vi "Device-Tester.vi"() -> ()   [LabVIEW 2011]
uses:
  <vilib>/Instr/_visa.llb/VISA Configure Serial Port (Instr).vi
panel:
  out "Bytes at Port":u32
  out "String Received":string
  in  "String to Send":string
  out "ExecTime":u32
  in  "BaudRate":u32(ring) items=["9600"=9600, "115200"=65535]
  in  "VISA resource name":refnum<visa-resource-name>
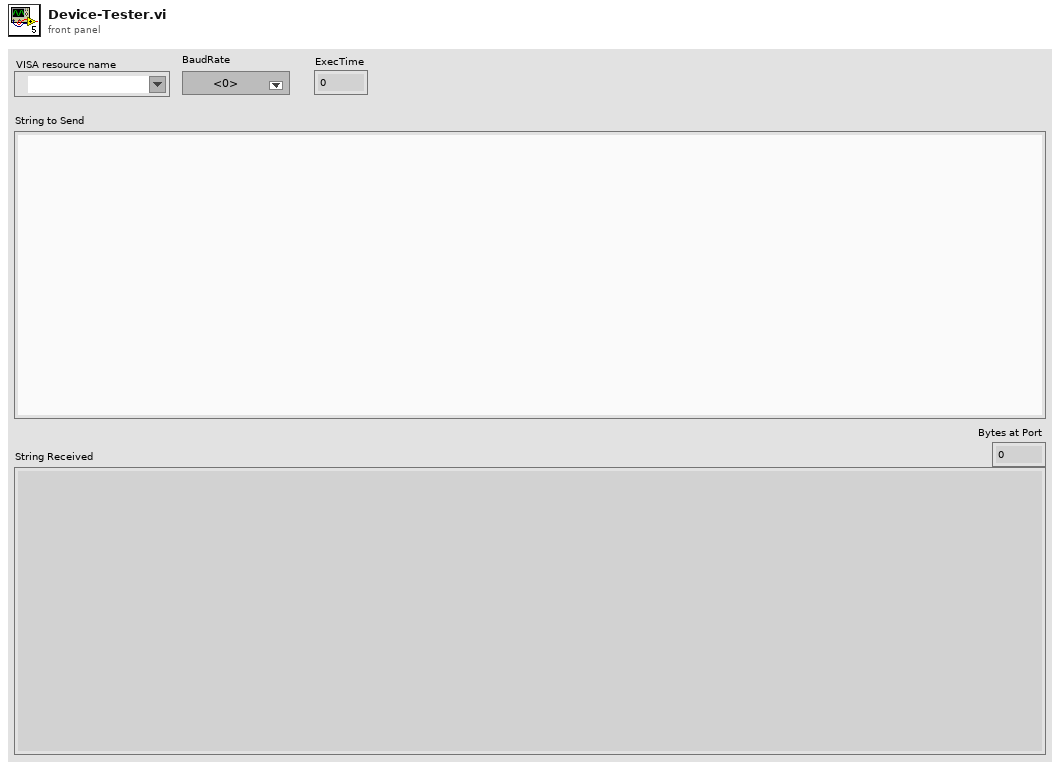
[diagram p1: front panel]
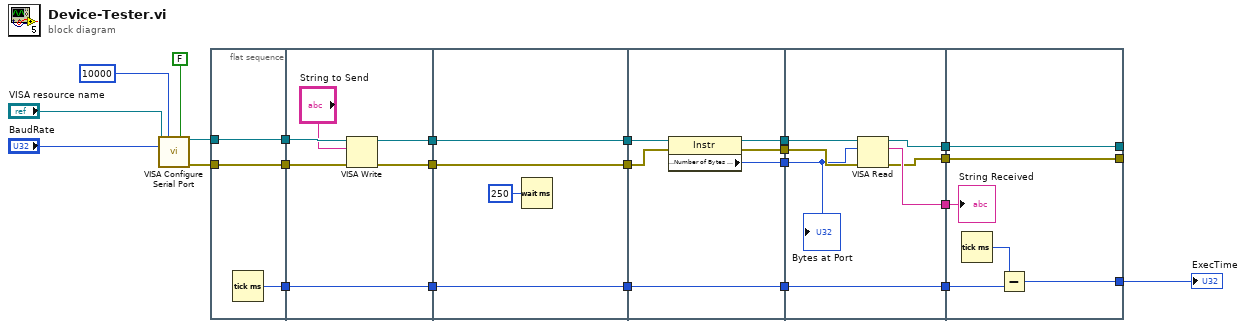
[diagram p0: block diagram]
diagram:
  n1 = call-poly "VISA Configure Serial Port"("VISA resource name"="VISA resource name", "timeout (10sec)"=u32 10000, "Enable Termination\nChar (T)"=FALSE ("Enable Termination\nChar (T)"), "baud rate (9600)"="BaudRate") -> ("VISA resource name out"=w20:refnum<visa-resource-name>, "error out"=w19:errorcluster)  [unwired: 10 in]
  n2 = flat-sequence {
    tunnel: w19 -> [w25]
    tunnel: w20 -> [w26]
    tunnel: [w26] -> w18
    tunnel: [w27] -> w17
    tunnel: [w25] -> w2
    tunnel: w18 -> [w32]
    tunnel: [w33] -> w9
    tunnel: w17 -> [w33]
    tunnel: [w30] -> w7
    tunnel: [w29] -> w5
    tunnel: w2 -> [w28]
    tunnel: w9 -> [w37]
    tunnel: [w37] -> w8
    tunnel: w7 -> [w36]
    tunnel: [w36] -> w6
    tunnel: w5 -> [w35]
    tunnel: [w35] -> w4
    tunnel: w8 -> [w43]
    tunnel: [w43] -> w12
    tunnel: w6 -> [w42]
    tunnel: w4 -> [w41]
    tunnel: [w40] -> w11
    tunnel: [w39] -> w10
    tunnel: [w38] -> w3
    tunnel: [w49] -> w16
    tunnel: [w44] -> w15
    tunnel: w12 -> [w50]
    tunnel: [w50] -> w14
    tunnel: [w45] -> w13
    tunnel: w11 -> [w48]
    tunnel: w10 -> [w47]
    tunnel: w3 -> [w46]
    tunnel: [w55] -> _
    tunnel: [w56] -> _
    tunnel: w16 -> [w56]
    tunnel: w15 -> [w55]
    tunnel: w14 -> [w53]
    tunnel: [w52] -> w1
    tunnel: w13 -> [w51]
    frame #0 {
      n3 = Tick Count (ms)() -> (millisecond timer value=w27:u32)
    }
    frame #1 {
      n4 = VISA Write(VISA resource name=w32, write buffer="String to Send", error in (no error)=w28) -> (VISA resource name out=w30:refnum<visa-resource-name>, error out=w29:errorcluster)  [unwired: 1 out]
    }
    frame #2 {
      n5 = Wait (ms)(milliseconds to wait=u32 250) -> ()  [unwired: 1 out]
    }
    frame #3 {
      n6 = property class="Instr"(reference=w42, error in=w41) -> (reference out=w40:refnum<visa-resource-name>, error out=w39:errorcluster, "Serial Settings:Number of Bytes at Serial Port"=w38:u32)
    }
    frame #4 {
      n7 = VISA Read(VISA resource name=w48, byte count=w46, error in (no error)=w47) -> (VISA resource name out=w49:refnum<visa-resource-name>, read buffer=w45:string, error out=w44:errorcluster)  [unwired: 1 out]
      "Bytes at Port" <- w46
    }
    frame #5 {
      n8 = Tick Count (ms)() -> (millisecond timer value=w54:u32)
      n9 = Subtract(x=w54, y=w53) -> (x-y=w52:u32)
      "String Received" <- w51
    }
  }
  "ExecTime" <- w1
